vi "Migrate Shared Dependencies.vi"(0 "Project path":path, 5 "Measurement path":path, 7 "Common dependencies":path[](array[path]), 11 "error in (no error)":errorcluster) -> (4 "Outside items":string[](array[string]), 6 "Library":T1[](array[typedef]), 15 "error out":errorcluster)   [LabVIEW 2021, in "Multiple Migrator.lvlib"]
uses:
  Multiple Migrator.lvlib
  controls/Library Info.ctl
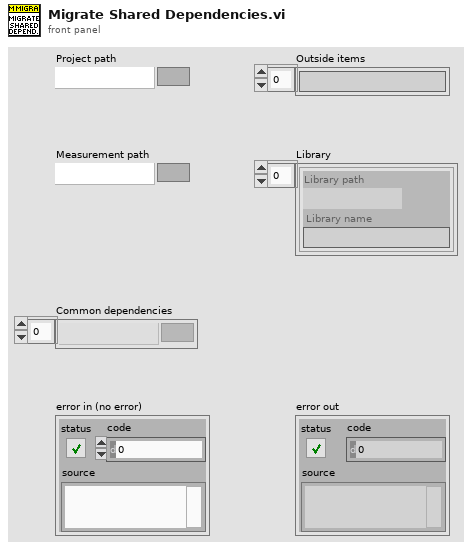
[diagram p1: front panel]
types:
  T1 = typedef "Multiple Migrator.lvlib/Library Info.ctl" = cluster{"Library path":path, "Library name":string}
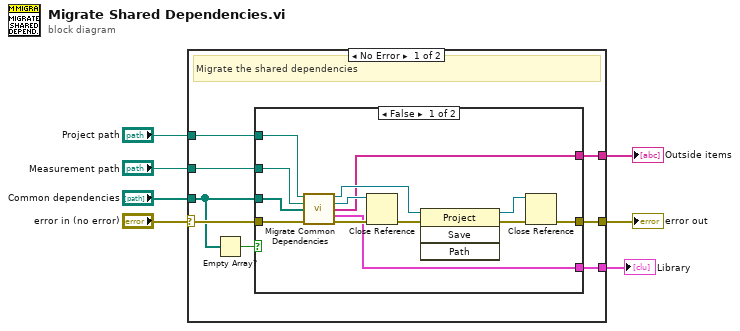
[diagram p0: block diagram]
diagram:
  n1 = case shown="No Error" "error in (no error)" {
    selector: "error in (no error)" -> [w14 w30]
    tunnel: [w15 w30] -> w7
    tunnel: "Common dependencies" -> [w11 _]
    tunnel: "Project path" -> [w13 _]
    tunnel: [w12 _] -> w3
    tunnel: "Measurement path" -> [w9 _]
    tunnel: [w8 _] -> w1
    frame No Error {
      # "Migrate the shared dependencies"
      n2 = Empty Array?(array=w11) -> (empty?=w10:bool)
      n3 = case shown="False" w10 {
        tunnel: w14 -> [w28 w29]
        tunnel: [w24 w29] -> w15
        tunnel: w11 -> [w20 _]
        tunnel: w13 -> [w19 _]
        tunnel: [w18 _] -> w12
        tunnel: w9 -> [w17 _]
        tunnel: [w16 _] -> w8
        frame False {
          n4 = call "Migrate Common Dependencies.vi"("Project path"=w19, "Measurement path"=w17, "Dependencies path"=w20, "error in (no error)"=w28) -> ("Project reference"=w22:refnum<vi>, "MeasurementCore reference"=w25:refnum<vi>, "Outside items"=w18:string[], "Library"=w16:T1[], "error out"=w27:errorcluster)  [unwired: 7 in]
          n5 = Close Reference(reference=w25, error in (no error)=w27) -> (error out=w26:errorcluster)
          n6 = invoke class="Project" method="Save"(reference=w22, error in=w26) -> (reference out=w21:refnum<vi>, error out=w23:errorcluster)  [unwired: 2 in, 2 out]
          n7 = Close Reference(reference=w21, error in (no error)=w23) -> (error out=w24:errorcluster)
        }
        frame True {
        }
      }
    }
    frame Error {
      # "Pass"
    }
  }
  "error out" <- w7
  "Outside items" <- w3
  "Library" <- w1
